vi "Script_Timing_Replace_Template_Values.vi"(8 "error in (no error)":errorcluster, 10 "Mandatory Items":T1={"Script Name"="ForTestPurpose", "GINI Time Period"=1000000.0, "HSDIO Delay"=60.0, "Shutter Duration before"=50000.0, "Shutter Duration after"=50000.0, "Filter Tau"=2000.0, "Trapping Delay"=600.0, "Trapping Duration"=300.0, "Emtyping Duration"=1000000.0} caption="TIMING Mandatory Items" {"GINI Time Period" min=100000.0 max=1000000.0 format="%#_7g"; "Shutter Duration after" min=2.0 max=100000.0; "HSDIO Delay" min=60.0 max=100.0; "Shutter Duration before" min=2.0 max=100000.0; "Filter Tau" min=1000.0 max=2000.0; "Trapping Delay" min=2.0; "Emtyping Duration" min=2.0 format="%#_8g"; "Trapping Duration" min=2.0}, 11 "Number of Ions Refills":i32=1 min=1 max=1000) -> (0 "error out":errorcluster, 3 "Ouput Script":string)   [LabVIEW 2018]
doc: "This VI replaces the macros strings of the template timing script by the TIMING Mandatory tems."
uses:
  controls/TIMING_Mandatory_Items.ctl
  controls/EXPERT_Path_Selector.ctl
panel:
  out "result string":string caption="chaîne résultante"
  in  "Chaîne":string
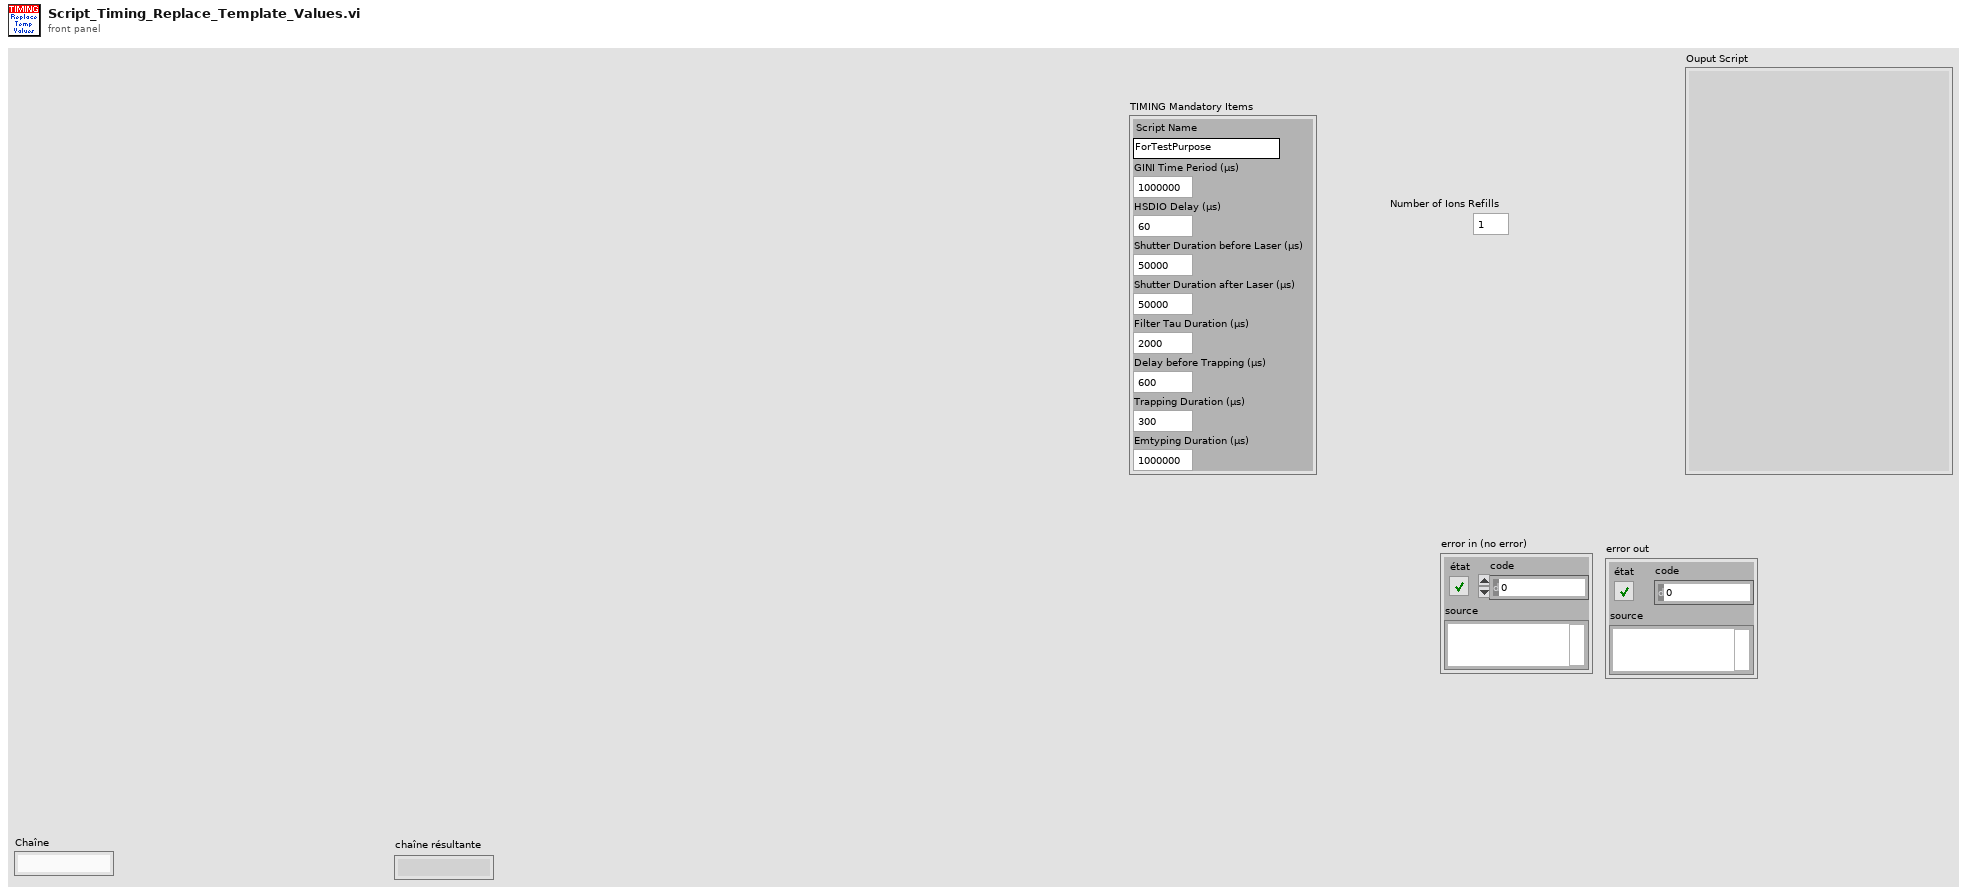
[diagram p1: front panel]
types:
  T1 = typedef "TIMING_Mandatory_Items.ctl" = cluster{"Script Name":string, "GINI Time Period":dbl, "HSDIO Delay":dbl, "Shutter Duration before":dbl, "Shutter Duration after":dbl, "Filter Tau":dbl, "Trapping Delay":dbl, "Trapping Duration":dbl, "Emtyping Duration":dbl}
  T2 = typedef "EXPERT_Path_Selector.ctl" = enum16{"Application", "Resources", "Data", "XML", "XML Saved", "Load Directory"}
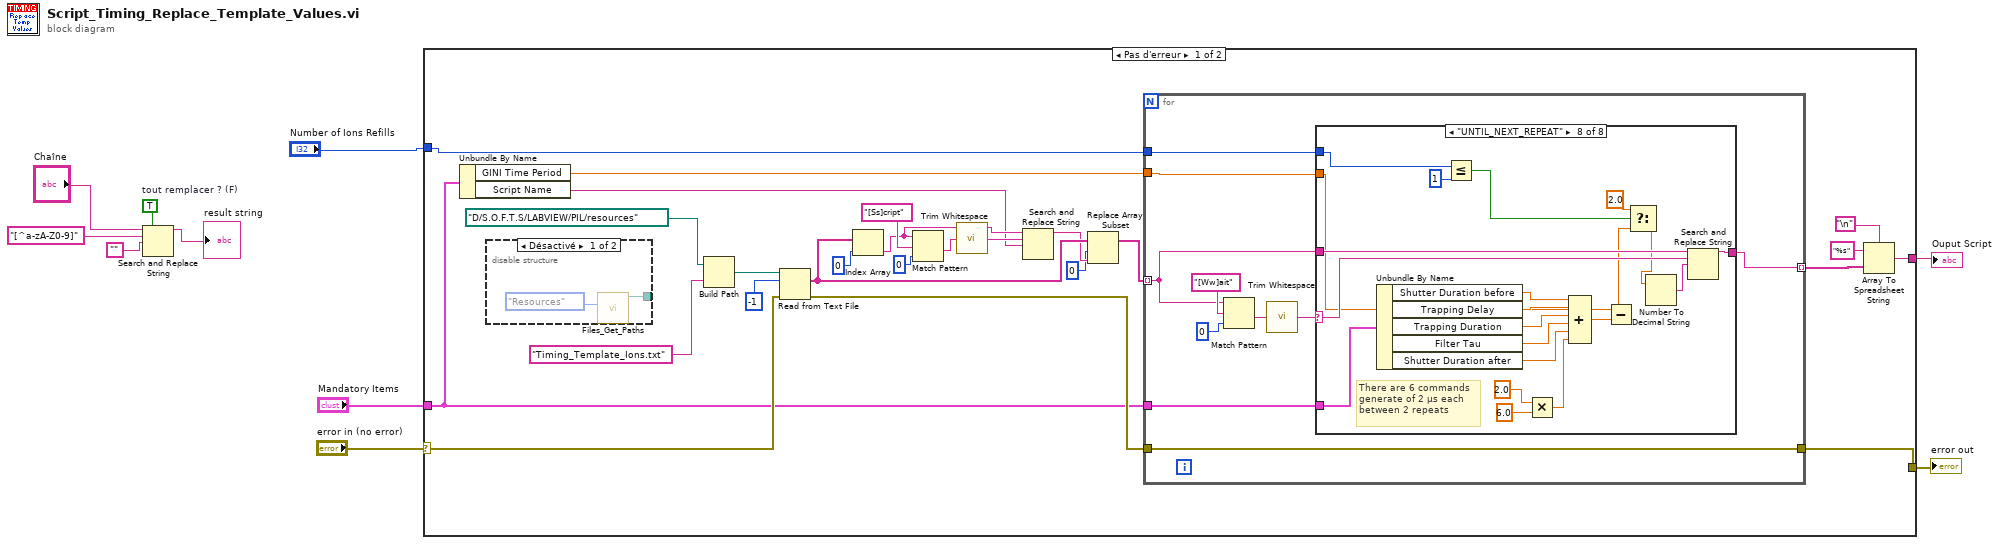
[diagram p0: block diagram]
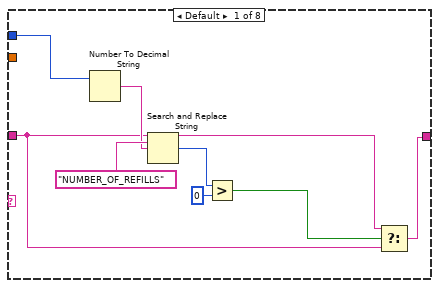
[diagram p3: hidden frame]
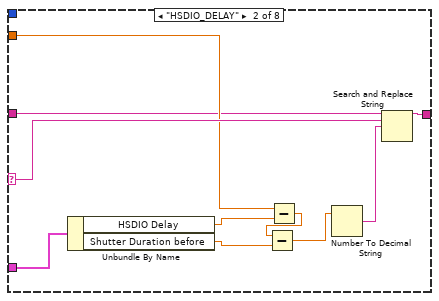
[diagram p4: hidden frame]
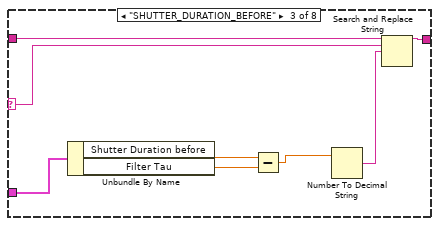
[diagram p5: hidden frame]
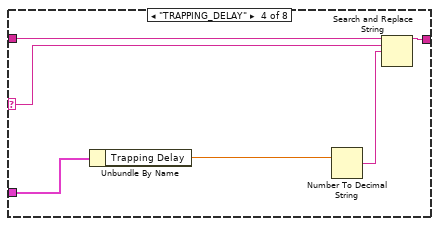
[diagram p6: hidden frame]
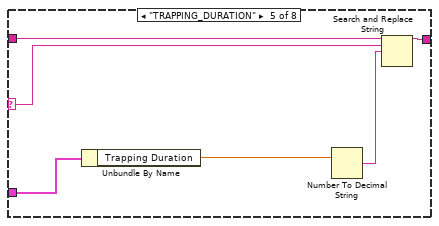
[diagram p7: hidden frame]
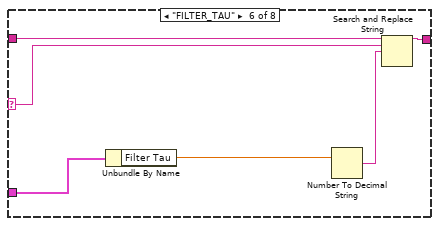
[diagram p8: hidden frame]
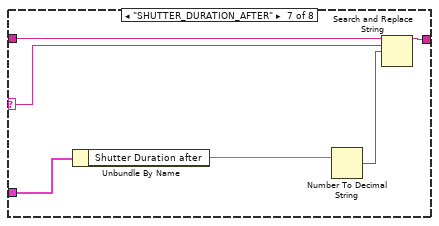
[diagram p9: hidden frame]
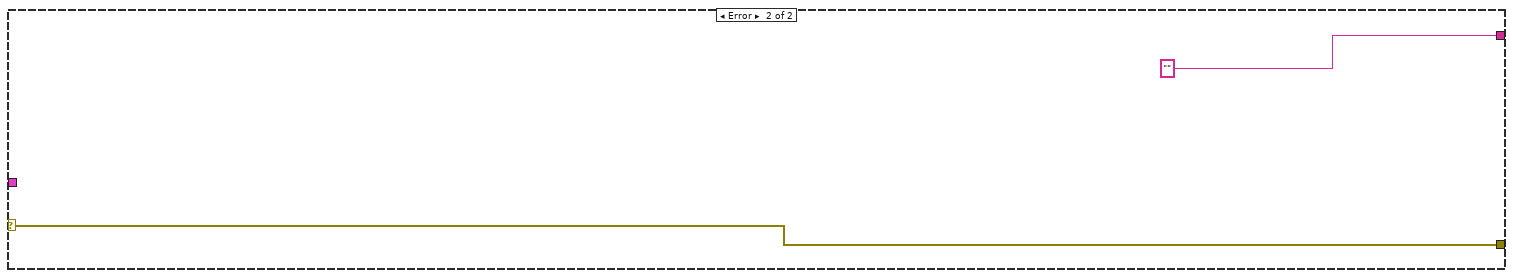
[diagram p10: hidden frame]
diagram:
  w1 = TRUE  # tout remplacer ? (F)
  n1 = Search and Replace String(replace all?=w1, input string="Chaîne", search string="[^a-zA-Z0-9]" ("regular expression (\"\")"), replace string="" ("replace string (\"\")")) -> (result string=→"result string":string)  [unwired: 4 in, 3 out]
  n2 = case shown="Pas d'erreur" "error in (no error)" {
    selector: "error in (no error)" -> [w32 w121]
    tunnel: [w31 w121] -> w9
    tunnel: "Mandatory Items" -> [w24 _]
    tunnel: [w27 "" ("spreadsheet string")] -> w7
    tunnel: "Number of Ions Refills" -> [w25 _]
    frame No Error {
      n3 = Unbundle By Name(w24) -> ("GINI Time Period"=w23:dbl, "Script Name"=w16:string)
      n4 = disable-structure shown="Désactivé" {
        disable-tunnel: [w36 _] -> _
        frame Disabled {
          n5 = call "Files_Get_Paths.vi"("EXPERT Path Selector"=EXPERT_Path_Selector."Resources") -> ("Path"=w36:path)  [unwired: 9 in, 1 out]
        }
        frame Enabled {
        }
      }
      n6 = Build Path(base path=path "D:/S.O.F.T.S/LABVIEW/PIL/resources" ("Path"), name or relative path="Timing_Template_Ions.txt" ("nom ou chemin relatif")) -> (appended path=w34:path)
      n7 = Read from Text File(file (use dialog)=w34, count=-1 ("nombre"), error in=w32) -> (text=w15:string[], error out=w30:errorcluster)  [unwired: 1 in, 2 out]
      n8 = Index Array(array=w15, index=0 ("indice")) -> (element=w17:string)
      n9 = Match Pattern(string=w17, regular expression="[Ss]cript" ("expression régulière"), offset (0)=0) -> (after substring=w19:string)  [unwired: 3 out]
      n10 = call <vilib>:"Trim Whitespace.vi"("string"=w19) -> ("trimmed string"=w18:string)  [unwired: 1 in]
      n11 = Search and Replace String(input string=w17, search string=w18, replace string=w16) -> (result string=w14:string)  [unwired: 5 in, 3 out]
      n12 = Replace Array Subset(array=w15, new element=w14, index=0 ("indice")) -> (w12:string[])
      n13 = for {
        tunnel: w30 -> [w45]
        tunnel: [w45] -> w31
        tunnel: w24 -> [w43]
        tunnel: [w39] -> w29 mode=indexing
        tunnel: w23 -> [w42]
        tunnel: w25 -> [w40]
        tunnel: w12 -> [w38] mode=indexing
        n14 = Match Pattern(string=w38, regular expression="[Ww]ait", offset (0)=0) -> (after substring=w46:string)  [unwired: 3 out]
        n15 = call <vilib>:"Trim Whitespace.vi"("string"=w46) -> ("trimmed string"=w44:string)  [unwired: 1 in]
        n16 = case shown="\"UNTIL_NEXT_REPEAT\"" w44 {
          selector: w44 -> [_ w65 w73 w79 w85 w91 w97 w118]
          tunnel: w43 -> [_ w66 w74 w80 w86 w92 w98 w119]
          tunnel: [w53 w64 w72 w78 w84 w90 w96 w117] -> w39
          tunnel: w42 -> [_ w58 _ _ _ _ _ w100]
          tunnel: w40 -> [w52 _ _ _ _ _ _ w105]
          tunnel: w38 -> [w48 w57 w67 w75 w81 w87 w93 w106]
          frame Default {
            n17 = Number To Decimal String(number=w52) -> (decimal integer string=w51:string)  [unwired: 1 in]
            n18 = Search and Replace String(input string=w48, search string="NUMBER_OF_REFILLS" ("chaîne recherchée"), replace string=w51) -> (result string=w49:string, number of replacements=w50:i32)  [unwired: 5 in, 2 out]
            n19 = Greater?(x=w50, y=0) -> (0:w54:bool)
            n20 = Select(t=w49, s=w54, f=w48) -> (s? t:f=w53:string)
          }
          frame "HSDIO_DELAY" {
            n21 = Unbundle By Name(w66) -> ("HSDIO Delay"=w63:dbl, "Shutter Duration before"=w60:dbl)
            n22 = Subtract(x=w58, y=w63) -> (x-y=w61:dbl)
            n23 = Subtract(x=w61, y=w60) -> (x-y=w59:dbl)
            n24 = Number To Decimal String(number=w59) -> (decimal integer string=w62:string)  [unwired: 1 in]
            n25 = Search and Replace String(input string=w57, search string=w65, replace string=w62) -> (result string=w64:string)  [unwired: 5 in, 3 out]
          }
          frame "SHUTTER_DURATION_BEFORE" {
            n26 = Unbundle By Name(w74) -> ("Shutter Duration before"=w70:dbl, "Filter Tau"=w69:dbl)
            n27 = Subtract(x=w70, y=w69) -> (x-y=w68:dbl)
            n28 = Number To Decimal String(number=w68) -> (decimal integer string=w71:string)  [unwired: 1 in]
            n29 = Search and Replace String(input string=w67, search string=w73, replace string=w71) -> (result string=w72:string)  [unwired: 5 in, 3 out]
          }
          frame "TRAPPING_DELAY" {
            n30 = Unbundle By Name(w80) -> ("Trapping Delay"=w76:dbl)
            n31 = Number To Decimal String(number=w76) -> (decimal integer string=w77:string)  [unwired: 1 in]
            n32 = Search and Replace String(input string=w75, search string=w79, replace string=w77) -> (result string=w78:string)  [unwired: 5 in, 3 out]
          }
          frame "TRAPPING_DURATION" {
            n33 = Unbundle By Name(w86) -> ("Trapping Duration"=w82:dbl)
            n34 = Number To Decimal String(number=w82) -> (decimal integer string=w83:string)  [unwired: 1 in]
            n35 = Search and Replace String(input string=w81, search string=w85, replace string=w83) -> (result string=w84:string)  [unwired: 5 in, 3 out]
          }
          frame "FILTER_TAU" {
            n36 = Unbundle By Name(w92) -> ("Filter Tau"=w88:dbl)
            n37 = Number To Decimal String(number=w88) -> (decimal integer string=w89:string)  [unwired: 1 in]
            n38 = Search and Replace String(input string=w87, search string=w91, replace string=w89) -> (result string=w90:string)  [unwired: 5 in, 3 out]
          }
          frame "SHUTTER_DURATION_AFTER" {
            n39 = Unbundle By Name(w98) -> ("Shutter Duration after"=w94:dbl)
            n40 = Number To Decimal String(number=w94) -> (decimal integer string=w95:string)  [unwired: 1 in]
            n41 = Search and Replace String(input string=w93, search string=w97, replace string=w95) -> (result string=w96:string)  [unwired: 5 in, 3 out]
          }
          frame "UNTIL_NEXT_REPEAT" {
            # "There are 6 commands\ngenerate of 2 µs each\nbetween 2 repeats"
            n42 = Unbundle By Name(w119) -> ("Shutter Duration before"=w111:dbl, "Trapping Delay"=w115:dbl, "Trapping Duration"=w114:dbl, "Filter Tau"=w113:dbl, "Shutter Duration after"=w112:dbl)
            n43 = Less Or Equal?(x=w105, y=1) -> (x <= y?=w103:bool)
            n44 = Multiply(x=2.0, y=6.0) -> (x*y=w107:dbl)
            n45 = Compound Arithmetic op=ADD(w111, w115, w114, w113, w112, w107) -> (w110:dbl)
            n46 = Subtract(x=w100, y=w110) -> (x-y=w99:dbl)
            n47 = Select(t=2.0 ("cas vrai"), s=w103, f=w99) -> (s? t:f=w101:dbl)
            n48 = Number To Decimal String(number=w101) -> (decimal integer string=w116:string)  [unwired: 1 in]
            n49 = Search and Replace String(input string=w106, search string=w118, replace string=w116) -> (result string=w117:string)  [unwired: 5 in, 3 out]
          }
        }
      }
      n50 = Array To Spreadsheet String(delimiter (Tab)="\n", array=w29, 3:"%s" ("chaîne de format")) -> (spreadsheet string=w27:string)
    }
    frame Error {
    }
  }
  "error out" <- w9
  "Ouput Script" <- w7
